vi "Read Plugin Configuration.vi"(8 "error in (no error)":errorcluster, 9 "Plugin File Path":path, 10 "Plugin Details in":T4, 11 "Refnum in":T3) -> (0 "error out":errorcluster, 2 "Plugin Details out":T4, 3 "refnum out":T3)   [LabVIEW 2020, in "RxnRover.lvlib" / "Plugin Manager.lvlib"]
doc: "Reads .conf (configuration file) included for each plugin while also checking if the .conf file is valid, then fills that information into an array of plugin details. If there are any invalid entries within the .conf file an error message with the specifc cause and a debug message is added to the Config Error cluster within plugin details. Logging is dealt with later in other VI's (Filter Invalid Plugins.vi , Log Plugin Errors.vi etc.)"
uses:
  Plugin Manager.lvlib
  Plugin Details.ctl
  Plugin Servers/Controller/Controller Type.ctl
  Plugin Types.ctl
  Config Error.ctl
  <vilib>/Utility/config.llb/Config Data RefNum.ctl
  <vilib>/Utility/config.llb/Read Key (String).vi
  <vilib>/Utility/config.llb/Read Key (Path).vi
  <vilib>/Utility/config.llb/NI_LVConfig.lvlib
  Plugin Servers/Controller/Generic Plugin.lvclass
  logging/logging.lvlib
panel:
  in  "Controller Type":T1
  in  "Plugin Type":T2
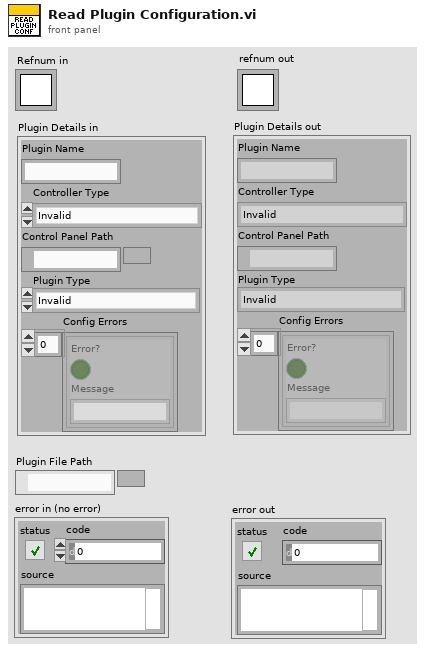
[diagram p1: front panel]
types:
  T1 = typedef "RxnRover.lvlib/Generic Plugin.lvclass/Controller Type.ctl" = enum16{"Invalid", "Temperature Controller", "Pump Controller", "Syringe Pump", "Generic Optimizer", "LC Parser", "Passive Hardware"}
  T2 = typedef "RxnRover.lvlib/Plugin Manager.lvlib/Plugin Types.ctl" = enum16{"Invalid", "Optimizer", "Analyzer", "Hardware"}
  T3 = typedef "NI_LVConfig.lvlib/Config Data RefNum.ctl" = refnum<k1>
  T4 = typedef "RxnRover.lvlib/Plugin Manager.lvlib/Plugin Details.ctl" = cluster{"Plugin Name":string, "Controller Type":T1, "Control Panel Path":path, "Plugin Type":T2, "Config Errors":T5[]}
  T5 = typedef "RxnRover.lvlib/Plugin Manager.lvlib/Config Error.ctl" = cluster{"Error?":bool, "Message":string}
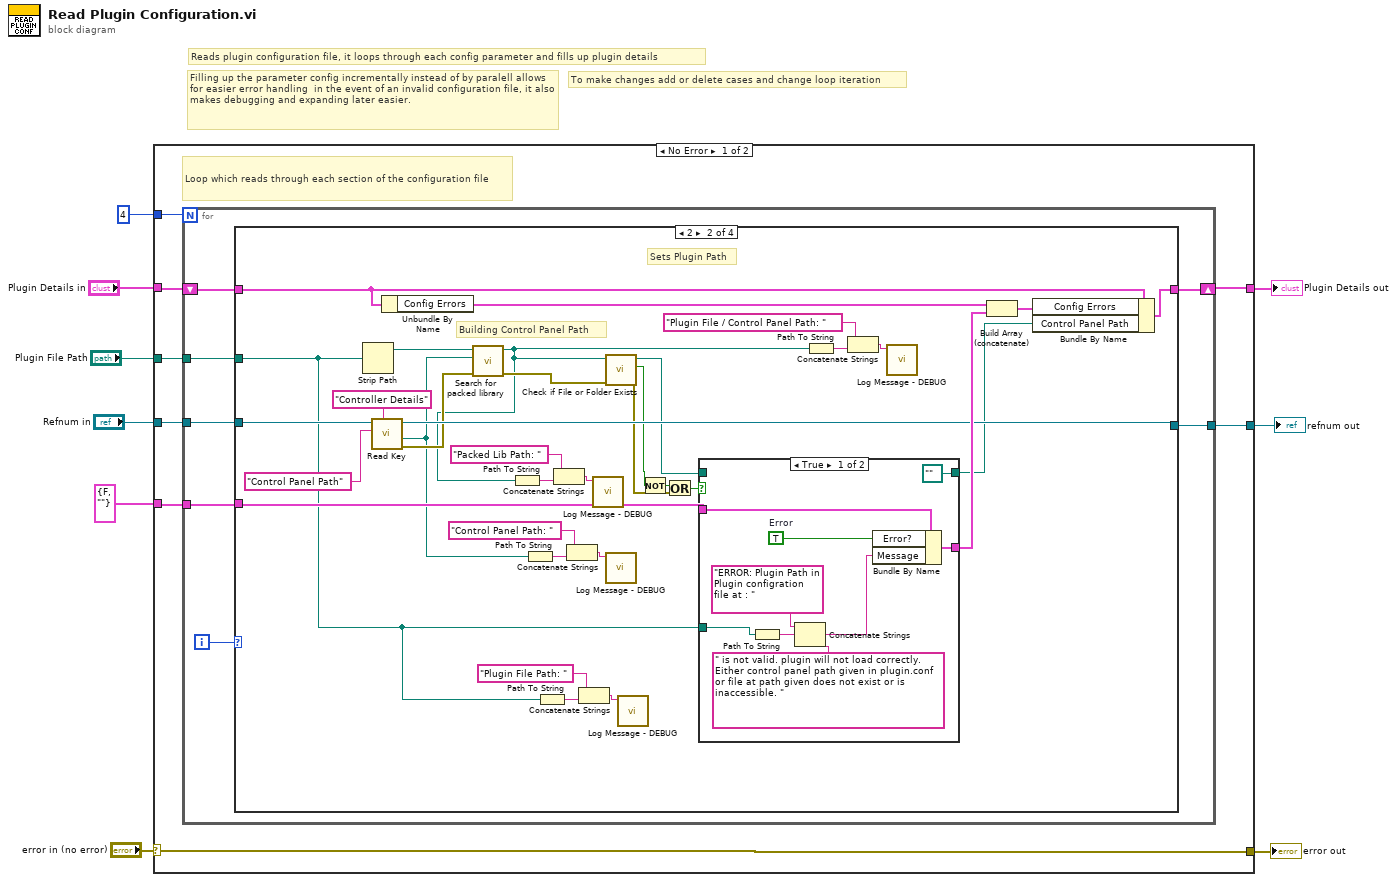
[diagram p0: block diagram]
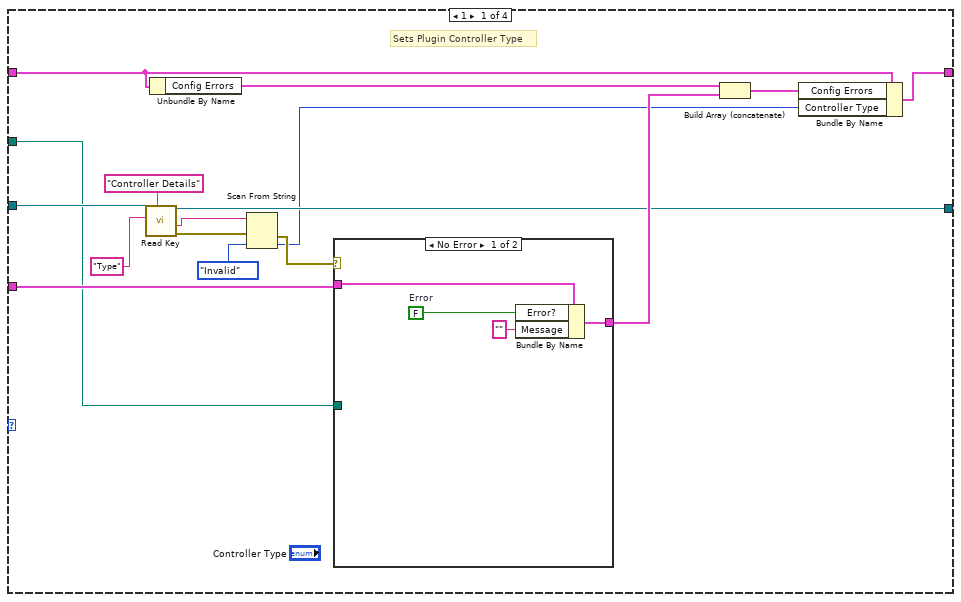
[diagram p2: hidden frame]
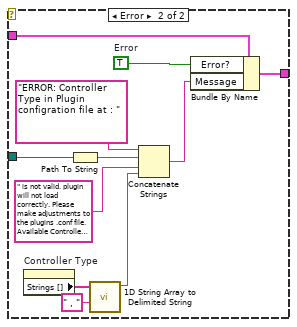
[diagram p3: hidden frame]
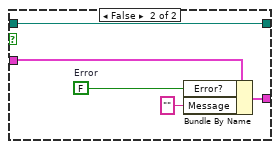
[diagram p4: hidden frame]
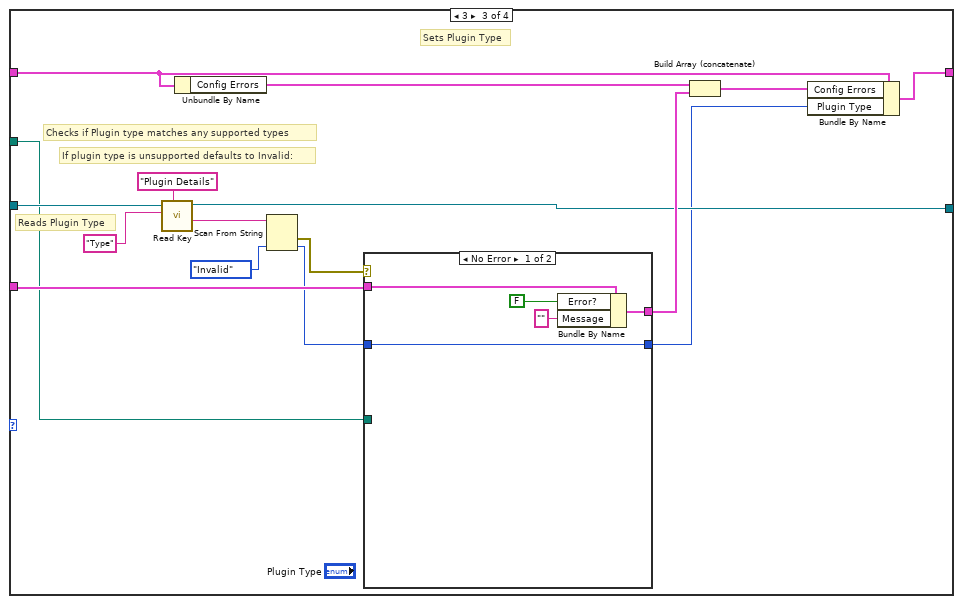
[diagram p5: hidden frame]
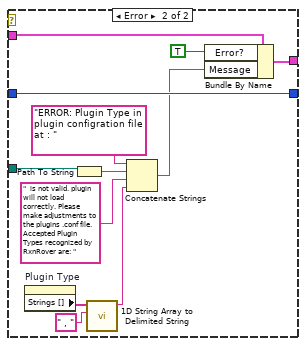
[diagram p6: hidden frame]
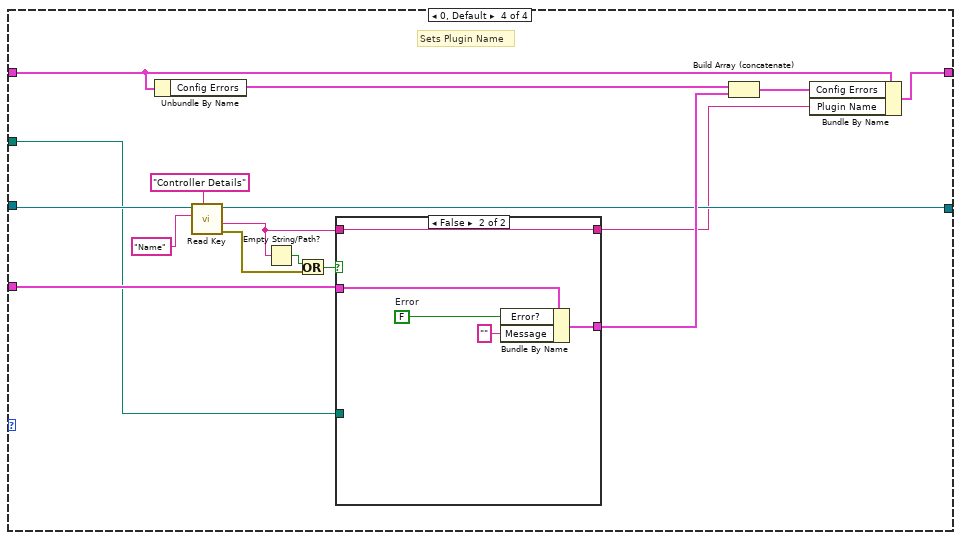
[diagram p7: hidden frame]
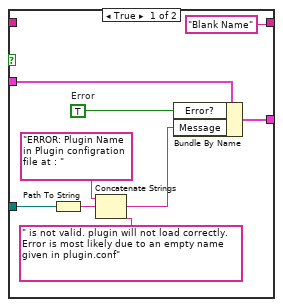
[diagram p8: hidden frame]
diagram:
  # "To make changes add or delete cases and change loop iteration"
  # "Filling up the parameter config incrementally instead of by paralell allows for easier error handling  in the event of an invalid configuration file, it also makes debugging and expanding later easier."
  # "Reads plugin configuration file, it loops through each config parameter and fills up plugin details"
  n1 = case shown="No Error" "error in (no error)" {
    selector: "error in (no error)" -> [w13 w167]
    tunnel: "Plugin Details in" -> [w17 w168]
    tunnel: [w15 w168] -> w8
    tunnel: [w14 w169] -> w7
    tunnel: "Refnum in" -> [w16 w169]
    tunnel: [w13 w167] -> w1
    tunnel: "Plugin File Path" -> [w12 _]
    tunnel: T5 {"Error?"=FALSE, "Message"=""} ("Config Error") -> [w11 _]
    tunnel: 4 -> [w10 _]
    frame No Error {
      # "Loop which reads through each section of the configuration file"
      n2 = for {
        N: w10 -> [_]
        tunnel: w16 -> [w22]
        tunnel: w12 -> [w21]
        tunnel: [w19] -> w14
        shift-right: [w20] -> w15
        shift-left: w17 -> [w24]
        tunnel: w11 -> [w18]
        i -> [w23]
        n3 = case shown="2" w23 {
          tunnel: w24 -> [w38 w87 w118 w150]
          tunnel: w18 -> [w39 w88 w111 w151]
          tunnel: [w30 w84 w117 w147] -> w20
          tunnel: w22 -> [w33 w83 w112 w146]
          tunnel: w21 -> [w32 w57 w108 w145]
          tunnel: [w31 w82 w109 w144] -> w19
          frame 1 {
            # "Sets Plugin Controller Type"
            n4 = call-poly <vilib>:"Read Key.vi"("section"="Controller Details", "key"="Type", "refnum"=w33) -> ("error out"=w35:errorcluster, "value"=w34:string, "refnum out"=w31:T3)  [unwired: 5 in, 1 out]
            n5 = Unbundle By Name(w38) -> ("Config Errors"=w36:T5[])
            n6 = Scan From String(input string=w34, error in=w35, default 1=Controller_Type."Invalid" ("Controller Type")) -> (error out=w28:errorcluster, output 1=w26:T1)  [unwired: 2 in, 2 out]
            n7 = case shown="No Error" w28 {
              tunnel: w32 -> [_ w49]
              tunnel: w39 -> [w44 w50]
              tunnel: [w42 w51] -> w37
              frame No Error {
                w43 = FALSE  # Error
                n8 = Bundle By Name(cluster=w44, "Error?"=w43, "Message"="") -> (w42:T5)
              }
              frame Error {
                w53 = TRUE  # Error
                n9 = property on="Controller Type" class="Enum (strict)"() -> ("Strings []"=w47:string[])  [unwired: 2 in, 2 out]
                n10 = Path To String(path=w49) -> (string=w55:string)
                n11 = call <vilib>:"1D String Array to Delimited String.vi"("delimiter"=" , ", "string array"=w47) -> ("delimited string"=w45:string)  [unwired: 9 in]
                n12 = Concatenate Strings("ERROR: Controller Type in Plugin configration file at : ", w55, " is not valid. plugin will not load correctly. Please make adjustments to the plugins .conf file. Available Controller Types recognized by RxnRover are: ", w45) -> (w52:string)
                n13 = Bundle By Name(cluster=w50, "Error?"=w53, "Message"=w52) -> (w51:T5)
              }
            }
            n14 = Build Array (concatenate)(w36, w37) -> (w27:T5[])
            n15 = Bundle By Name(cluster=w38, "Config Errors"=w27, "Controller Type"=w26) -> (w30:T4)
          }
          frame 2 {
            # "Building Control Panel Path"
            # "Sets Plugin Path"
            n16 = Strip Path(path=w57) -> (stripped path=w56:path)  [unwired: 1 out]
            n17 = call-poly <vilib>:"Read Key.vi"("section"="Controller Details", "key"="Control Panel Path", "refnum"=w83) -> ("error out"=w74:errorcluster, "value"=w61:path, "refnum out"=w82:T3)  [unwired: 5 in, 1 out]
            n18 = Unbundle By Name(w87) -> ("Config Errors"=w85:T5[])
            n19 = call "Search for packed library.vi"("error in (no error)"=w74, "Control Panel Path"=w61, "Plugin Directory Path"=w56) -> ("error out (no error)"=w73:errorcluster, "Control Panel Path Out"=w65:path)  [unwired: 7 in]
            n20 = Path To String(path=w65) -> (string=w68:string)
            n21 = Path To String(path=w61) -> (string=w64:string)
            n22 = Path To String(path=w57) -> (string=w60:string)
            n23 = Concatenate Strings("Packed Lib Path: " ("string"), w68) -> (w67:string)
            n24 = Concatenate Strings("Control Panel Path: " ("string"), w64) -> (w63:string)
            n25 = Concatenate Strings("Plugin File Path: " ("string"), w60) -> (w59:string)
            n26 = call "Log Message - DEBUG.vi"("Message"=w67) -> ()  [unwired: 10 in, 1 out]
            n27 = call <vilib>:"Check if File or Folder Exists.vi"("error in (no error)"=w73, "path"=w65) -> ("error out"=w78:errorcluster, "file or folder exists?"=w76:bool, "dup path"=w72:path)  [unwired: 7 in]
            n28 = call "Log Message - DEBUG.vi"("Message"=w63) -> ()  [unwired: 10 in, 1 out]
            n29 = call "Log Message - DEBUG.vi"("Message"=w59) -> ()  [unwired: 10 in, 1 out]
            n30 = Not(x=w76) -> (.not. x?=w75:bool)
            n31 = Or(x=w75, y=w78) -> (x .or. y?=w79:bool)
            n32 = case shown="True" w79 {
              tunnel: w57 -> [w92 _]
              tunnel: w88 -> [w93 w103]
              tunnel: [w94 w101] -> w86
              tunnel: w72 -> [_ w99]
              tunnel: [path "" ("dup path") w99] -> w77
              frame True {
                w96 = TRUE  # Error
                n33 = Path To String(path=w92) -> (string=w98:string)
                n34 = Concatenate Strings("ERROR: Plugin Path in Plugin configration file at : ", w98, " is not valid. plugin will not load correctly. Either control panel path given in plugin.conf or file at path given does not exist or is inaccessible. ") -> (w95:string)
                n35 = Bundle By Name(cluster=w93, "Error?"=w96, "Message"=w95) -> (w94:T5)
              }
              frame False {
                w102 = FALSE  # Error
                n36 = Bundle By Name(cluster=w103, "Error?"=w102, "Message"="") -> (w101:T5)
              }
            }
            n37 = Path To String(path=w65) -> (string=w71:string)
            n38 = Concatenate Strings("Plugin File / Control Panel Path: " ("string"), w71) -> (w70:string)
            n39 = call "Log Message - DEBUG.vi"("Message"=w70) -> ()  [unwired: 10 in, 1 out]
            n40 = Build Array (concatenate)(w85, w86) -> (w80:T5[])
            n41 = Bundle By Name(cluster=w87, "Config Errors"=w80, "Control Panel Path"=w77) -> (w84:T4)
          }
          frame 3 {
            # "If plugin type is unsupported defaults to Invalid:"
            # "Checks if Plugin type matches any supported types"
            # "Reads Plugin Type"
            # "Sets Plugin Type"
            n42 = call-poly <vilib>:"Read Key.vi"("section"="Plugin Details", "key"="Type", "refnum"=w112) -> ("value"=w116:string, "refnum out"=w109:T3)  [unwired: 5 in, 2 out]
            n43 = Unbundle By Name(w118) -> ("Config Errors"=w119:T5[])
            n44 = Scan From String(input string=w116, default 1=Plugin_Types."Invalid" ("Plugin Type")) -> (error out=w113:errorcluster, output 1=w104:T2)  [unwired: 3 in, 2 out]
            n45 = case shown="No Error" w113 {
              tunnel: w104 -> [w124 w135]
              tunnel: [w124 w135] -> w106
              tunnel: [w122 w136] -> w110
              tunnel: w111 -> [w123 w134]
              tunnel: w108 -> [_ w129]
              frame No Error {
                n46 = Bundle By Name(cluster=w123, "Error?"=FALSE, "Message"="") -> (w122:T5)
              }
              frame Error {
                n47 = property on="Plugin Type" class="Enum (strict)"() -> ("Strings []"=w125:string[])  [unwired: 2 in, 2 out]
                n48 = Path To String(path=w129) -> (string=w132:string)
                n49 = call <vilib>:"1D String Array to Delimited String.vi"("delimiter"=" , ", "string array"=w125) -> ("delimited string"=w126:string)  [unwired: 9 in]
                n50 = Concatenate Strings("ERROR: Plugin Type in plugin configration file at : ", w132, "  is not valid. plugin will not load correctly. Please make adjustments to the plugins .conf file. Accepted Plugin Types recognized by RxnRover are: ", w126) -> (w128:string)
                n51 = Bundle By Name(cluster=w134, "Error?"=TRUE, "Message"=w128) -> (w136:T5)
              }
            }
            n52 = Build Array (concatenate)(w119, w110) -> (w107:T5[])
            n53 = Bundle By Name(cluster=w118, "Config Errors"=w107, "Plugin Type"=w106) -> (w117:T4)
          }
          frame 0, Default {
            # "Sets Plugin Name"
            n54 = Unbundle By Name(w150) -> ("Config Errors"=w148:T5[])
            n55 = call-poly <vilib>:"Read Key.vi"("section"="Controller Details", "key"="Name", "refnum"=w146) -> ("error out"=w140:errorcluster, "value"=w138:string, "refnum out"=w144:T3)  [unwired: 5 in, 1 out]
            n56 = Empty String/Path?(string/path=w138) -> (empty?=w139:bool)
            n57 = Or(x=w139, y=w140) -> (x .or. y?=w141:bool)
            n58 = case shown="False" w141 {
              tunnel: w145 -> [w154 _]
              tunnel: w151 -> [w156 w166]
              tunnel: [w157 w164] -> w149
              tunnel: w138 -> [_ w162]
              tunnel: ["Blank Name" ("value") w162] -> w137
              frame True {
                w159 = TRUE  # Error
                n59 = Path To String(path=w154) -> (string=w161:string)
                n60 = Concatenate Strings("ERROR: Plugin Name in Plugin configration file at : ", w161, " is not valid. plugin will not load correctly. Error is most likely due to an empty name given in plugin.conf") -> (w158:string)
                n61 = Bundle By Name(cluster=w156, "Error?"=w159, "Message"=w158) -> (w157:T5)
              }
              frame False {
                w165 = FALSE  # Error
                n62 = Bundle By Name(cluster=w166, "Error?"=w165, "Message"="") -> (w164:T5)
              }
            }
            n63 = Build Array (concatenate)(w148, w149) -> (w142:T5[])
            n64 = Bundle By Name(cluster=w150, "Config Errors"=w142, "Plugin Name"=w137) -> (w147:T4)
          }
        }
      }
    }
    frame Error {
    }
  }
  "Plugin Details out" <- w8
  "error out" <- w1
  "refnum out" <- w7
